vi "Actor Core.vi"(8 "error in":errorcluster, 11 "BoundViewManager In":refnum<class "BoundViewManager.lvclass">=refnum) -> (0 "error out":errorcluster, 3 "Actor out":refnum<class "Actor.lvclass">)   [LabVIEW 2020, in "BoundViewManager.lvlib" / "BoundViewManager.lvclass"]
doc: "(<B>Filename</B>: Actor Framework.lvlib:Actor.lvclass:Actor Core.vi)\n\nReceives messages to the actor, reacts to them, and initiates any error handling that may shut the actor down.\n\nDescendant classes may override this VI to append parallel tasks for the actor to complete while it handles messages. Overrides use the Call Parent Method node.\n\n<License>\nCopyright © 2017 Composed Systems, LLC | All rights reserved\nwww.composed.io\n\nAuthor: Ethan Stern <ethan.stern@composed.io>\n\nThis software is provided \"AS IS\" WITHOUT WARRANTIES, either express or implied, AND IS FOR EDUCATIONAL PURPOSES ONLY.\n</License>"
uses:
  BoundViewManager.lvclass
  modules/mva-viewable/Source/IViewable/ProtectedSubpanel/ProtectedSubpanel.lvclass
  modules/mva-viewable/Source/IViewManager/IViewManager/IViewManager.lvclass
  <vilib>/ActorFramework/Actor/Actor.lvclass
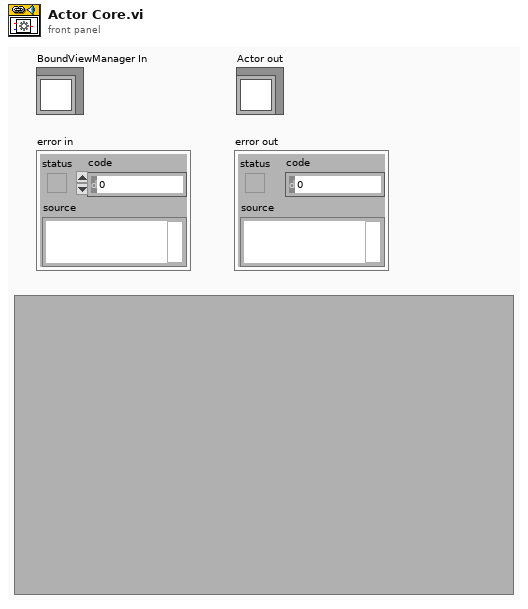
[diagram p1: front panel]
types:
  T1 = typedef "IViewable.lvlib/ProtectedSubpanel.lvclass/Protected Subpanel Reference.ctl" = refnum<data-value>
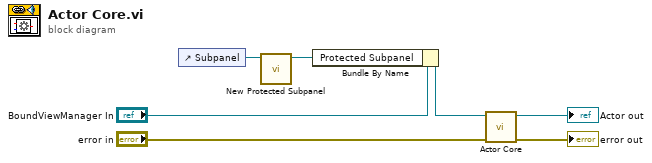
[diagram p0: block diagram]
diagram:
  n1 = control-ref of="Subpanel"() -> (w1:refnum<vi>)
  n2 = call "New Protected Subpanel.vi"("SubPnl Refnum"=w1) -> ("Protected Subpanel"=w2:T1)  [unwired: 9 in, 1 out]
  n3 = Bundle By Name(cluster="BoundViewManager In", "Protected Subpanel"=w2) -> (w3:refnum<class "BoundViewManager.lvclass">)
  n4 = call-parent "Actor Core.vi"("error in"="error in", "IViewable In"=w3) -> ("error out"=→"error out":errorcluster, "Actor out"=→"Actor out":refnum<class "Actor.lvclass">)  [unwired: 8 in]
